vi "Read_Temperature.vi"() -> ()   [LabVIEW 2021]
uses:
  <vilib>/DAQmx/create/channels.llb/DAQmx Create Channel (AI-Voltage-Basic).vi
  <vilib>/Analysis/NI_AALBase.lvlib
  <vilib>/DAQmx/configure/timing.llb/DAQmx Timing (Sample Clock).vi
  <vilib>/DAQmx/read.llb/DAQmx Read (Analog 1D DBL 1Chan NSamp).vi
  <vilib>/Analysis/baseanly.llb/Mean (DBL).vi
panel:
  out "Temp":dbl
  in  "Stop":bool
  out "Temp [Graph]":dbl(graph)
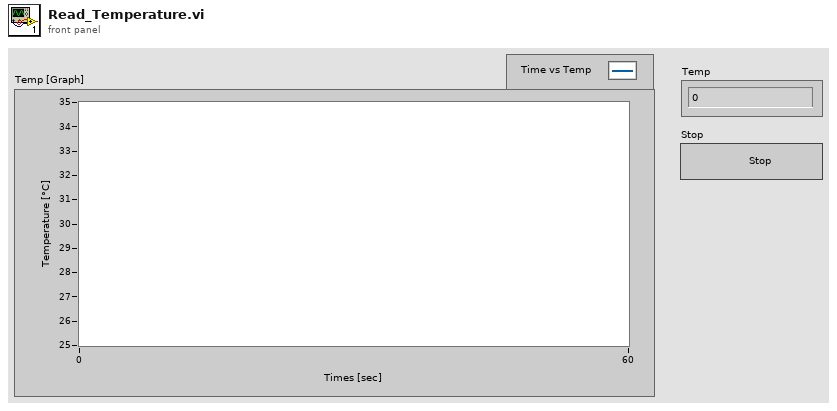
[diagram p1: front panel]
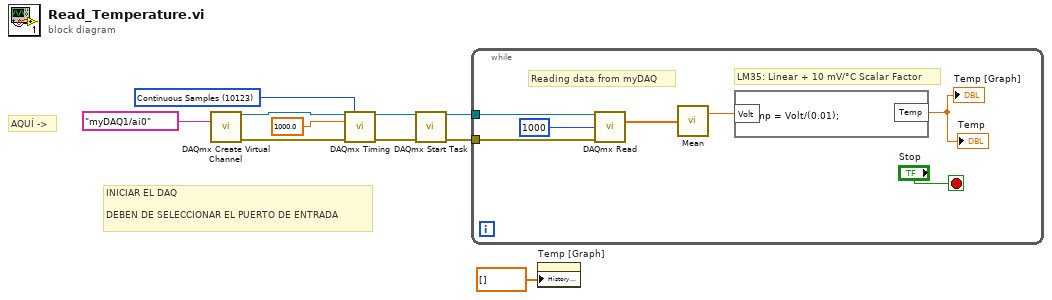
[diagram p0: block diagram]
diagram:
  w9 = 10123 items=["Finite Samples"=10178, "Continuous Samples"=10123, "Hardware Timed Single Point"=12522] ("sample mode")
  # "AQUÍ ->"
  # "INICIAR EL DAQ\n\nDEBEN DE SELECCIONAR EL PUERTO DE ENTRADA"
  n1 = call-poly <vilib>:"DAQmx Create Virtual Channel.vi"("physical channels"=tag "myDAQ1/ai0") -> ("task out"=w3:refnum<k21>, "error out"=w2:errorcluster)  [unwired: 13 in]
  n2 = call-poly <vilib>:"DAQmx Timing.vi"("task/channels in"=w3, "sample mode"=w9, "rate"=1000.0, "error in"=w2) -> ("task out"=w7:refnum<k21>, "error out"=w6:errorcluster)  [unwired: 10 in]
  n3 = call <vilib>:"DAQmx Start Task.vi"("task/channels in"=w7, "error in"=w6) -> ("task out"=w5:refnum<k21>, "error out"=w4:errorcluster)  [unwired: 12 in]
  n4 = while {
    tunnel: w5 -> [w17]
    tunnel: w4 -> [w16]
    stop <- "Stop" stop-if-true
    # "Reading data from myDAQ"
    # "LM35: Linear + 10 mV/°C Scalar Factor"
    n5 = call-poly <vilib>:"DAQmx Read.vi"("task/channels in"=w17, "number of samples per channel"=1000, "error in"=w16) -> ("data"=w15:dbl[])  [unwired: 10 in, 2 out]
    n6 = call-poly <vilib>:"Mean.vi"("X"=w15) -> ("mean"=w14:dbl)  [unwired: 1 out]
    n7 = formula code="Temp = Volt/(0.01);"("Volt"=w14) -> ("Temp"=→"Temp" →"Temp [Graph]":dbl)
  }
  n8 = property on="Temp [Graph]" class="WFChart (strict)"("History Data"=dbl[] []) -> ()  [unwired: 2 in, 2 out]
